vi "Get Host to Target DMAMap.vi"(8 "error in (no error)":errorcluster, 11 "Item Ref in":T4 format="%.0x") -> (0 "error out":errorcluster, 2 "DMA configuration array":T1[](array[typedef]), 3 "Item Ref out":T4 format="%.0x")   [LabVIEW 2016, in "FPGA Addon System Explorer.lvlib"]
uses:
  FPGA Addon System Explorer.lvlib
  <vilib>/NI Veristand/Custom Device API/Custom Device Item Ref.ctl
  <vilib>/rvi/FIFO/Fifo_Types/Fifo_DMA_Config.ctl
  <vilib>/rvi/DataTransferAndStorage/Container/Common/niFpgaDataTypeControl.ctl
  <vilib>/rvi/ClientSDK/Core/ModuleGeneration/CommunicationInterfaceUtility/niFpgaDmaChannelImplementation.ctl
  <vilib>/NI Veristand/Custom Device API/Get Item Property (Variant).vi
  Shared/Constants.vi
  Shared/FPGA Addon Shared.lvlib
  <vilib>/NI VeriStand/Custom Device API/Custom Device API.lvlib
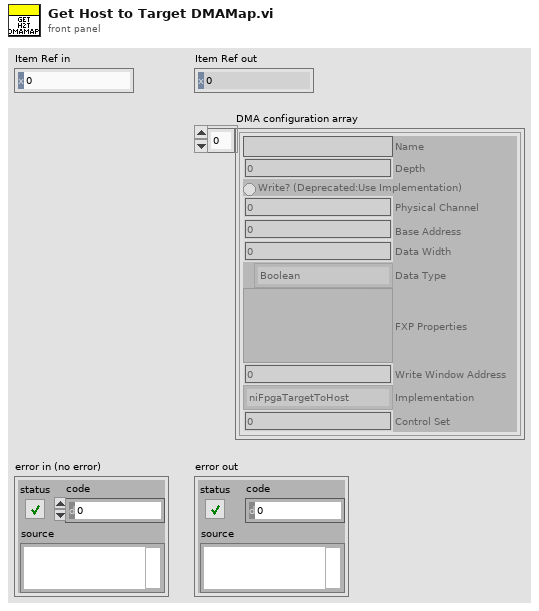
[diagram p1: front panel]
types:
  T1 = typedef "Fifo_DMA_Config.ctl" = cluster{"Name":string, "Depth":u32, "Write? (Deprecated:Use Implementation)":bool, "Physical Channel":u32, "Base Address":u32, "Data Width":u32, "Data Type":T2, "FXP Properties":variant, "Write Window Address":u32, "Implementation":T3, "Control Set":u32}
  T2 = typedef "niFpgaDataTypeControl.ctl" = enum32{"Boolean", "I8", "I16", "I32", "I64", "U8", "U16", "U32", "U64", "FXP", "CustomControl", "SGL"}
  T3 = typedef "niFpgaDmaChannelImplementation.ctl" = enum16{"niFpgaTargetToHost", "niFpgaHostToTarget", "niFpgaPeerToPeerWriter", "niFpgaPeerToPeerReader", "niCoreTargetToHost", "niCoreHostToTarget"}
  T4 = typedef "Custom Device API.lvlib/Custom Device Item Ref.ctl" = u64
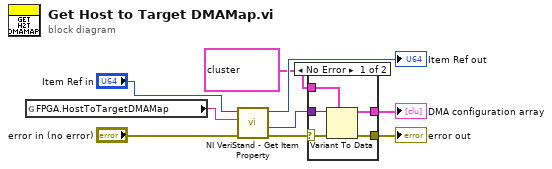
[diagram p0: block diagram]
diagram:
  n1 = global read "Constants.vi" "FPGA.HostToTargetDMAMap"() -> (w8:string)
  n2 = call-poly <vilib>:"NI VeriStand - Get Item Property.vi"("error in (no error)"="error in (no error)", "Property Name"=w8, "Item Ref in"="Item Ref in") -> ("error out"=w4:errorcluster, "Value"=w5:variant, "Item Ref out"=→"Item Ref out":T4)  [unwired: 5 in, 1 out]
  n3 = case shown="No Error" w4 {
    selector: w4 -> [w12 w15]
    tunnel: [w14 w16] -> w1
    tunnel: w5 -> [w13 _]
    tunnel: [w11 w15] -> w3
    tunnel: T1[] [{"Name"="P2PSource", "Depth"=1023, "Write? (Deprecated:Use Implementation)"=TRUE, "Physical Channel"=0, "Base Address"=65472, "Data Width"=32, "Data Type"=enum."U32", "FXP Properties"=variant(fxp<+,32,32> 0.0), "Write Window Address"=0, "Implementation"=enum."niFpgaPeerToPeerWriter", "Control Set"=0}, {"Name"="P2PSink", "Depth"=1023, "Write? (Deprecated:Use Implementation)"=FALSE, "Physical Channel"=1, "Base Address"=65408, "Data Width"=32, "Data Type"=enum."U32", "FXP Properties"=variant(fxp<+,32,32> 0.0), "Write Window Address"=57344, "Implementation"=enum."niFpgaPeerToPeerReader", "Control Set"=1}] ("DMA configuration array") -> [w10 w16]
    frame No Error {
      n4 = Variant To Data(error in=w12, type=w10, Variant=w13) -> (data=w14:T1[], error out=w11:errorcluster)
    }
    frame Error {
    }
  }
  "error out" <- w3
  "DMA configuration array" <- w1
